vi "错误日志.vi"(11 "错误数组":errorcluster[](array[cluster])) -> (0 "错误信息数组":string[](array[string]), 3 "错误代码数组":i32[](array[numeric]))   [LabVIEW 2017]
uses:
  <vilib>/Utility/file.llb/Write To Spreadsheet File (string).vi
panel:
  in  "错误时间数组":string[](array[string])
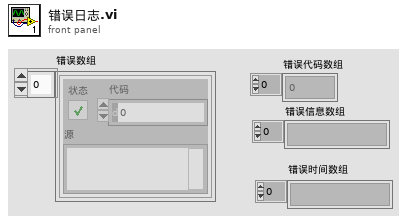
[diagram p1: front panel]
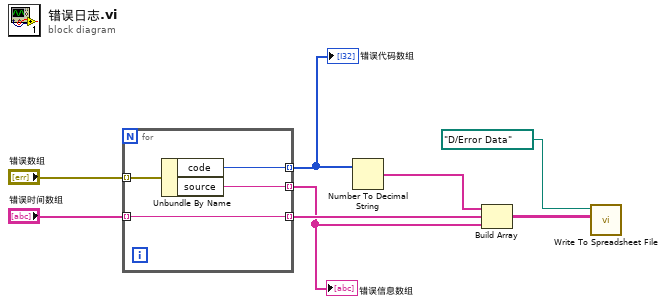
[diagram p0: block diagram]
diagram:
  n1 = for {
    tunnel: "错误数组" -> [w12] mode=indexing
    tunnel: [w11] -> w7 mode=indexing
    tunnel: [w10] -> w1 mode=indexing
    tunnel: "错误时间数组" -> [w9] mode=indexing
    tunnel: [w9] -> w2 mode=indexing
    n2 = Unbundle By Name(w12) -> ("code"=w11:i32, "source"=w10:string)
  }
  "错误代码数组" <- w7
  "错误信息数组" <- w1
  n3 = Number To Decimal String(number=w7) -> (decimal integer string=w6:string[])  [unwired: 1 in]
  n4 = Build Array(w6, w2, w1) -> (w5:string[][])
  n5 = call-poly <vilib>:"Write To Spreadsheet File.vi"("2D data"=w5, "file path (dialog if empty)"=path "D:/Error Data") -> ()  [unwired: 6 in, 1 out]
